vi "Adquisicio_projecte_InsEl.vi"() -> ()   [LabVIEW 2014]
uses:
  <vilib>/DAQmx/read.llb/DAQmx Read.vi
  <vilib>/DAQmx/read.llb/DAQmx Read (Analog 1D Wfm NChan NSamp).vi
  <vilib>/DAQmx/create/channels.llb/DAQmx Create Channel (AI-Voltage-Basic).vi
  <vilib>/DAQmx/configure/timing.llb/DAQmx Timing (Sample Clock).vi
  <vilib>/DAQmx/miscellaneous.llb/DAQmx Fill In Error Info.vi
panel:
  in  "stop":bool
  out "data":waveform(dbl)[](graph)
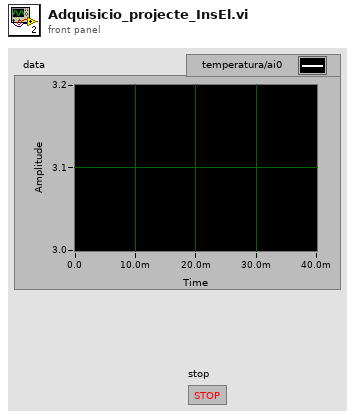
[diagram p1: front panel]
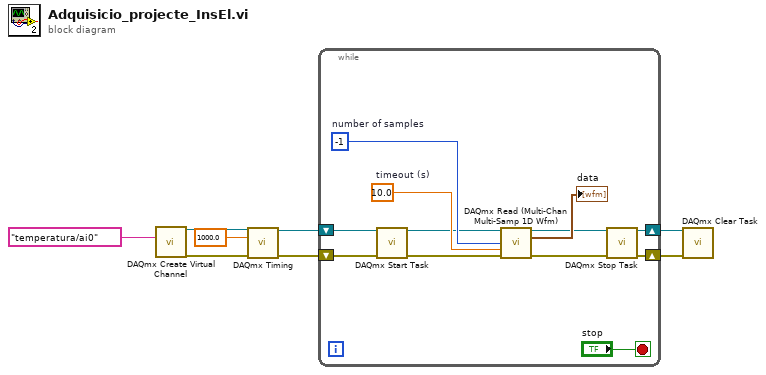
[diagram p0: block diagram]
diagram:
  n1 = call-poly <vilib>:"DAQmx Create Virtual Channel.vi"("physical channels"=tag "temperatura/ai0") -> ("task out"=w3:refnum<k21>, "error out"=w4:errorcluster)  [unwired: 13 in]
  n2 = call-poly <vilib>:"DAQmx Timing.vi"("task/channels in"=w3, "rate"=1000.0, "error in"=w4) -> ("task out"=w6:refnum<k21>, "error out"=w5:errorcluster)  [unwired: 11 in]
  n3 = while {
    shift-right: [w15] -> w8
    shift-left: w6 -> [w11]
    shift-right: [w14] -> w7
    shift-left: w5 -> [w10]
    stop <- "stop" stop-if-true
    w18 = 10.0  # timeout (s)
    w19 = -1  # number of samples
    n4 = call <vilib>:"DAQmx Start Task.vi"("task/channels in"=w11, "error in"=w10) -> ("task out"=w16:refnum<k21>, "error out"=w17:errorcluster)  [unwired: 12 in]
    n5 = call-poly "DAQmx Read (Multi-Chan Multi-Samp 1D Wfm).vi"("task/channels in"=w16, "number of samples per channel"=w19, "timeout"=w18, "error in"=w17) -> ("task out"=w13:refnum<k21>, "data"=→"data":waveform(dbl)[], "error out"=w12:errorcluster)  [unwired: 9 in]
    n6 = call <vilib>:"DAQmx Stop Task.vi"("task/channels in"=w13, "error in"=w12) -> ("task out"=w15:refnum<k21>, "error out"=w14:errorcluster)  [unwired: 12 in]
  }
  n7 = call <vilib>:"DAQmx Clear Task.vi"("task in"=w8, "error in"=w7) -> ()  [unwired: 13 in, 1 out]
